vi "Contour Line (Number of Heights).vi"(6 "number of heights":i32=10, 9 "Z":dbl[][](array[numeric]), 10 "Y":dbl[](array[numeric]), 11 "X":dbl[](array[numeric])) -> (0 "error":i32, 2 "Contour Line":T1[](array[typedef]), 3 "Contour Graph":cluster{dbl[], dbl[]}[](graph))   [LabVIEW 2017, in "NI_AAL_Geometry.lvlib"]
doc: "Calculates and returns the contour lines of a surface and the contour graph."
uses:
  <vilib>/Analysis/NI_AAL_Geometry.lvlib
  <vilib>/Analysis/geometry.llb/Contour Lines Control.ctl
  <vilib>/Analysis/geometry.llb/Contour Line Segment.ctl
  <vilib>/gmath/interp.llb/Create Mesh Grid (2D) (x,y arrays).vi
  <vilib>/gmath/NI_Gmath.lvlib
panel:
  # "Contour Line"
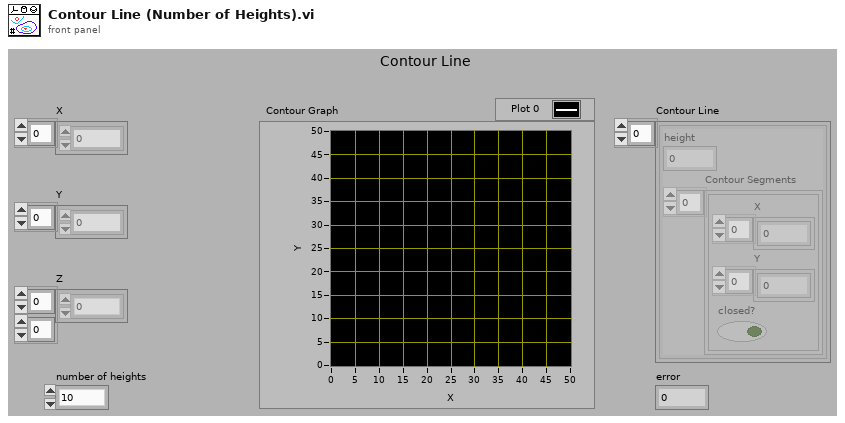
[diagram p1: front panel]
types:
  T1 = typedef "NI_AAL_Geometry.lvlib/Contour Lines Control.ctl" = cluster{"height":dbl, "Contour Segments":T2[]}
  T2 = typedef "NI_AAL_Geometry.lvlib/Contour Line Segment.ctl" = cluster{"X":dbl[], "Y":dbl[], "closed?":bool}
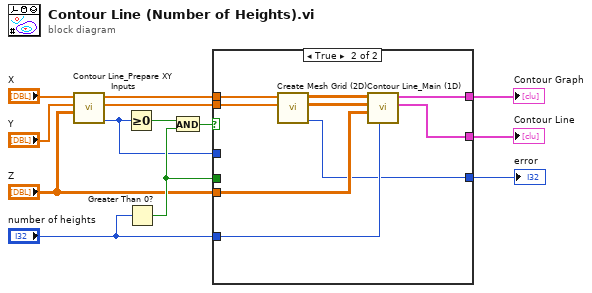
[diagram p0: block diagram]
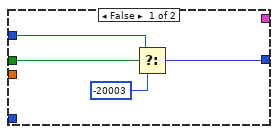
[diagram p2: hidden frame]
diagram:
  n1 = call <vilib>:"Contour Line_Prepare XY Inputs.vi"("Z In"="Z", "Y In"="Y", "X In"="X") -> ("error"=w1:i32, "Y Out"=w4:dbl[], "X Out"=w5:dbl[])  [unwired: 6 in]
  n2 = Greater Or Equal To 0?(x=w1) -> (x >= 0?=w2:bool)
  n3 = Greater Than 0?(x="number of heights") -> (x > 0?=w8:bool)
  n4 = And(x=w2, y=w8) -> (x .and. y?=w10:bool)
  n5 = case shown="True" w10 {
    tunnel: [_ w22] -> w13
    tunnel: w5 -> [_ w26]
    tunnel: "Z" -> [_ w23]
    tunnel: [_ w21] -> w12
    tunnel: [w15 w18] -> w11
    tunnel: w4 -> [_ w25]
    tunnel: "number of heights" -> [_ w19]
    tunnel: w8 -> [w17 _]
    tunnel: w1 -> [w14 _]
    frame False {
      n6 = Select(t=w14, s=w17, f=-20003) -> (s? t:f=w15:i32)
    }
    frame True {
      n7 = call-poly <vilib>:"Create Mesh Grid (2D).vi"("y domain"=w25, "x domain"=w26) -> ("error"=w18:i32, "Y"=w20:dbl[][], "X"=w24:dbl[][])  [unwired: 7 in]
      n8 = call <vilib>:"Contour Line_Main (1D).vi"("number of heights"=w19, "Z"=w23, "Y"=w20, "X"=w24) -> ("Contour Line"=w21:T1[], "Contour Graph"=w22:cluster{dbl[], dbl[]}[])  [unwired: 6 in]
    }
  }
  "error" <- w11
  "Contour Line" <- w12
  "Contour Graph" <- w13
